vi "Main.vi"(11 "Module Admin":refnum<class "Delacor_lib_QMH_Module Admin.lvclass">) -> ()   [LabVIEW 2020, in "Config.lvlib"]
doc: "This template is based off of the Queued Message Handler design pattern and the Queued Message Handler project template that ships with LabVIEW.\n\nThe main difference is that the queue is private to this module and communication between modules is performed via Broadcast and Request events.\n\nRequest events are wrapped in public API methods and are handled in the Event Handling Loop (EHL) of this VI. Any module can register for Broadcast events sent by this module. The EHL generates messages based on user interface actions.\n\nThe Message Handling Loop (MHL) processes messages generated by the EHL, or by other messages. The messages are string values, so new messages can be added easily to the Message Cases case structure in the MHL. Each message cluster can also provide an optional value for Message Data, which is a variant that can be converted to whatever message-specific data is required.\n_____\nBased on Delacor QMH Project Template 5.0.0.82."
uses:
  Config.lvlib
  <vilib>/Delacor/Delacor QMH/Libraries/Module Admin_class/Delacor_lib_QMH_Module Admin.lvclass
  Module Data--cluster.ctl
  Stop Argument--cluster.ctl
  <vilib>/Delacor/Delacor QMH/Libraries/Message Queue_class/Delacor_lib_QMH_Message Queue.lvclass/Delacor_lib_QMH_Message Queue.ctl
  <vilib>/Utility/miscctls.llb/LVPointTypeDef.ctl
  <vilib>/Delacor/Delacor QMH/Libraries/Module Admin_class/Delacor_lib_QMH_Module Admin.lvclass/Delacor_lib_QMH_Module Admin.ctl
  <vilib>/Delacor/Delacor QMH/Libraries/Message Queue_class/Delacor_lib_QMH_Enqueue Message (Single).vi
  <vilib>/Delacor/Delacor QMH/Libraries/Module Admin_class/Delacor_lib_QMH_Get External Launch.vi
  <vilib>/Utility/error.llb/Error Cluster From Error Code.vi
  <vilib>/ErrorRing/Error Ring.xnode
  <vilib>/Delacor/Delacor QMH/Libraries/Message Queue_class/Delacor_lib_QMH_Message Queue.lvclass
  Acquisition/Acquisition.lvlib
  Loggin/Loggin.lvlib
panel:
  in  "file name":string
  in  "Config":T1={"sampling info"={"Fs"=1000.0, "#s"=1000.0}, "square wave duty cycle (%)"=50.0, "frequency"=10.0, "amplitude"=1.0, "phase"=0.0, "signal type"=enum."Sine Wave"}
  out "error out":errorcluster
  out "Status":string
  # "Config"
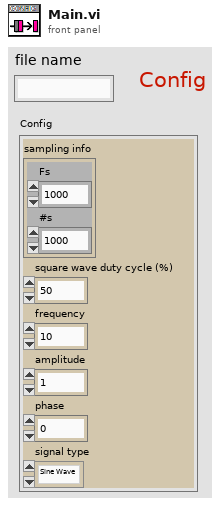
[diagram p1: front panel]
types:
  T1 = cluster{"sampling info":cluster{"Fs":dbl, "#s":dbl}, "square wave duty cycle (%)":dbl, "frequency":dbl, "amplitude":dbl, "phase":dbl, "signal type":enum16{"Sine Wave", "Triangle Wave", "Square Wave", "Sawtooth Wave"}}
  T2 = typedef "Config.lvlib/Request Events--cluster.ctl" = cluster{"Stop Module":refnum<user-event>, "Show Panel":refnum<user-event>, "Hide Panel":refnum<user-event>, "Get Module Execution Status":refnum<user-event>, "Show Diagram":refnum<user-event>}
  T3 = typedef "Config.lvlib/Module Data--cluster.ctl" = cluster{"Status":string}
  T4 = enum32{"invalid lock state", "Not Locked", "Locked (No Password)", "Password-protected"}
  T5 = typedef "Config.lvlib/Stop Argument--cluster.ctl" = cluster{"Origin":string, "Exit via Stop Module Req?":bool, "Wait for Module to stop?":bool}
  T6 = typedef "LVPointTypeDef.ctl" = cluster{"Horizontal":i16, "Vertical":i16}
  T7 = enum32{"Invalid", "Standard", "Closed", "Hidden", "Minimized", "Maximized"}
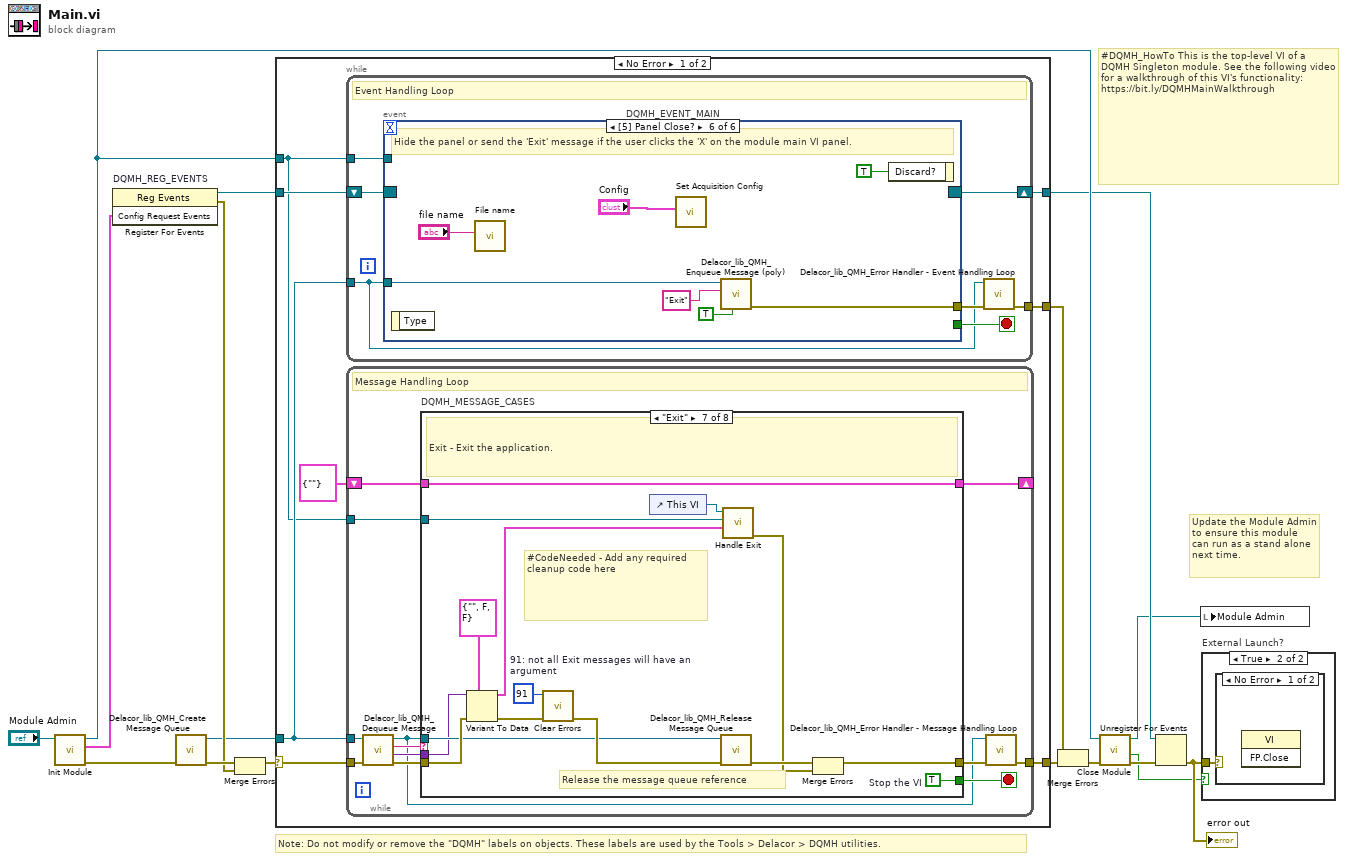
[diagram p0: block diagram]
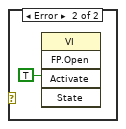
[diagram p3: hidden frame]
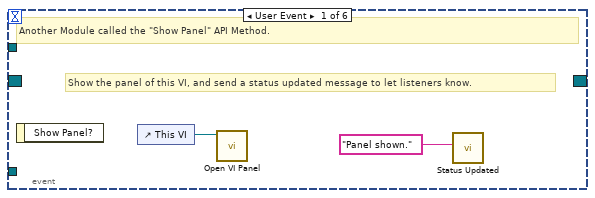
[diagram p4: hidden frame]
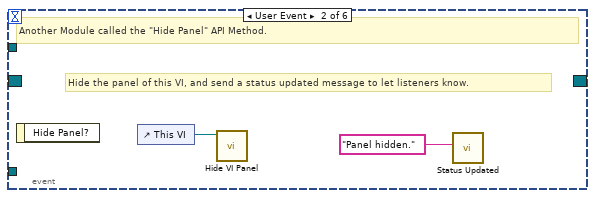
[diagram p5: hidden frame]
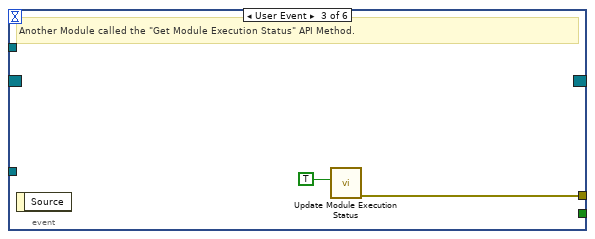
[diagram p6: hidden frame]
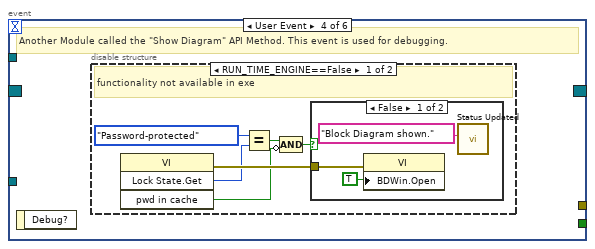
[diagram p7: hidden frame]
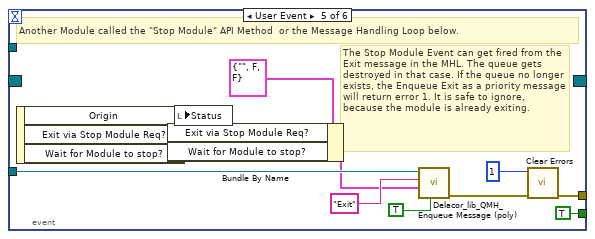
[diagram p10: hidden frame]
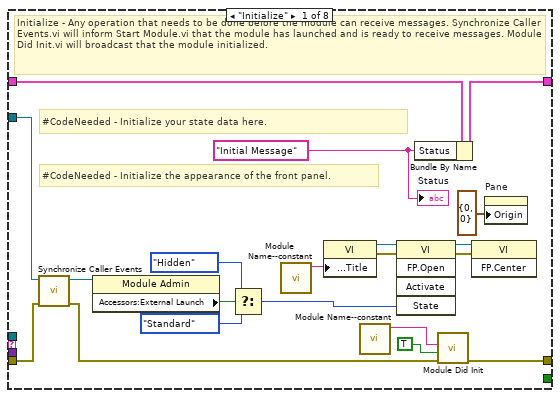
[diagram p11: hidden frame]
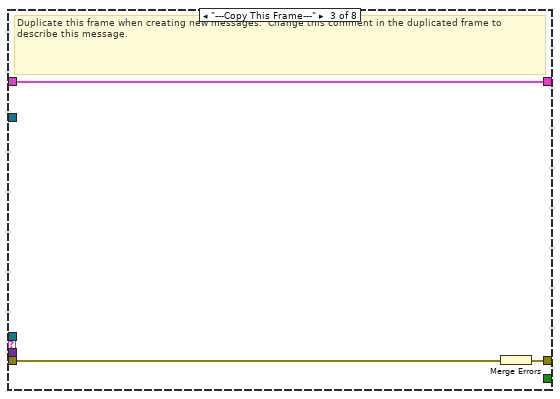
[diagram p13: hidden frame]
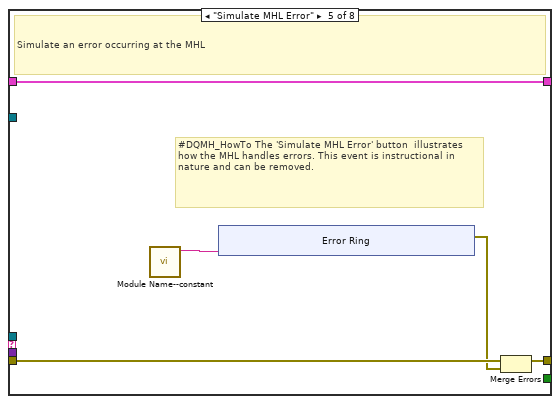
[diagram p15: hidden frame]
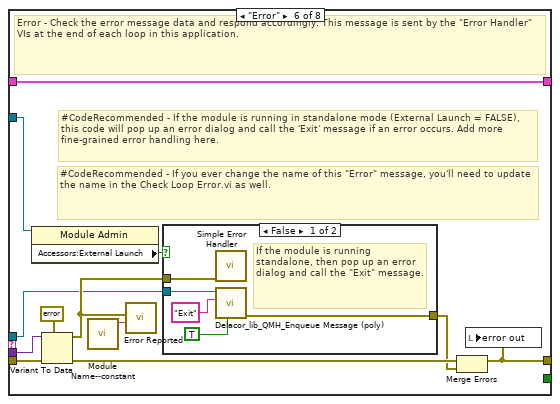
[diagram p16: hidden frame]
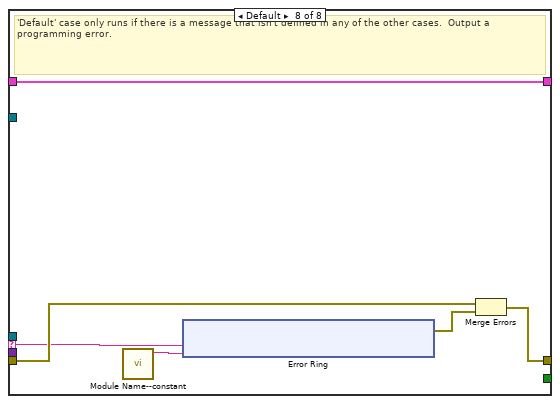
[diagram p18: hidden frame]
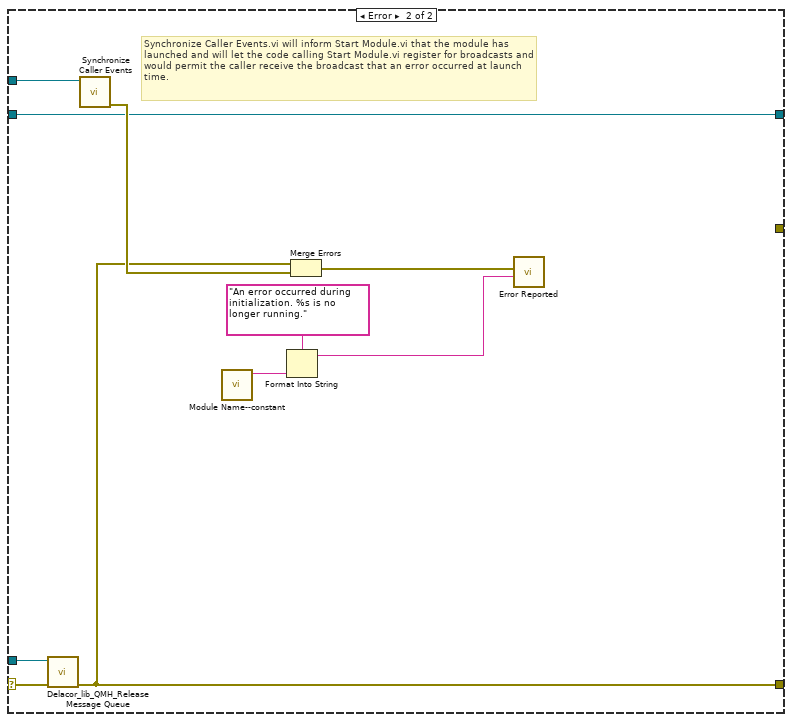
[diagram p19: hidden frame]
diagram:
  # "#DQMH_HowTo This is the top-level VI of a DQMH Singleton module. See the following video for a walkthrough of this VI's functionality: https://bit.ly/DQMHMainWalkthrough"
  # "Note: Do not modify or remove the \"DQMH\" labels on objects. These labels are used by the Tools > Delacor > DQMH utilities."
  # "Update the Module Admin to ensure this module can run as a stand alone next time."
  n1 = call "Init Module.vi"("Singleton Module Admin in"="Module Admin") -> ("error out"=w16:errorcluster, "Config Request Events"=w5:T2, "Singleton Module Admin out"=w8:refnum<class "Delacor_lib_QMH_Module Admin.lvclass">)  [unwired: 8 in]
  n2 = register-events "DQMH_REG_EVENTS"(w5) -> (reference out=w6:refnum<event-registration>, error out=w9:errorcluster)  [unwired: 2 in]
  n3 = call <vilib>:"Delacor_lib_QMH_Create Message Queue.vi"("error in (no error)"=w16) -> ("error out"=w11:errorcluster, "Message Queue"=w4:refnum<class "Delacor_lib_QMH_Message Queue.lvclass">)  [unwired: 9 in]
  n4 = Merge Errors(w11, w9) -> (w10:errorcluster)
  n5 = case shown="No Error" w10 {
    selector: w10 -> [w23 w166]
    tunnel: [w25 w165] -> w17
    tunnel: [w22 w171] -> w7
    tunnel: w6 -> [w20 w171]
    tunnel: w4 -> [w19 w164]
    tunnel: [w24 _] -> w14
    tunnel: w8 -> [w18 w167]
    frame No Error {
      n6 = while {
        tunnel: w19 -> [w26]
        shift-right: [w29] -> w22
        shift-left: w20 -> [w30]
        tunnel: [w31] -> w24
        tunnel: w18 -> [w27]
        stop <- w28 stop-if-true
        # "Event Handling Loop"
        n7 = event "DQMH_EVENT_MAIN" shown="[5] Panel Close?" {
          selector: w30 -> [_ _ _ _ _ _]
          dyn-events: [_ _ _ _ _ _] -> w29
          timeout: _ -> [_ _ _ _ _ _]
          tunnel: [_ _ _ _ TRUE ("Discard?") _] -> w28
          tunnel: w26 -> [_ _ _ _ w55 w64]
          tunnel: [_ _ w38 _ w58 w66] -> w32
          tunnel: w27 -> [_ _ _ _ _ _]
          event User Event {
            # "Show the panel of this VI, and send a status updated message to let listeners know."
            # "Another Module called the \"Show Panel\" API Method."
            n8 = event-data() -> ()  [unwired: 1 in, 1 out]
            n9 = control-ref of="This VI"() -> (w34:refnum<vi>)
            n10 = call "Open VI Panel.vi"("VI"=w34) -> ()  [unwired: 10 in, 1 out]
            n11 = call "Status Updated.vi"("Status"="Panel shown." ("format string")) -> ()  [unwired: 10 in, 1 out]
          }
          event User Event {
            # "Hide the panel of this VI, and send a status updated message to let listeners know."
            # "Another Module called the \"Hide Panel\" API Method."
            n12 = event-data() -> ()  [unwired: 1 in, 1 out]
            n13 = control-ref of="This VI"() -> (w36:refnum<vi>)
            n14 = call "Hide VI Panel.vi"("VI"=w36) -> ()  [unwired: 10 in, 1 out]
            n15 = call "Status Updated.vi"("Status"="Panel hidden." ("format string")) -> ()  [unwired: 10 in, 1 out]
          }
          event User Event {
            # "Another Module called the \"Get Module Execution Status\" API Method."
            n16 = event-data() -> ()  [unwired: 1 in, 1 out]
            n17 = call "Update Module Execution Status.vi"("Running?"=TRUE) -> ("error out"=w38:errorcluster)  [unwired: 10 in]
          }
          event User Event {
            # "Another Module called the \"Show Diagram\" API Method. This event is used for debugging."
            n18 = event-data() -> ()  [unwired: 1 in, 1 out]
            n19 = disable-structure shown="RUN_TIME_ENGINE==False" {
              frame condition #0 (active) {
                # "functionality not available in exe"
                n20 = invoke class="VI" method="Lock State.Get"() -> (error out=w44:errorcluster, "Get Lock State"=w43:T4, "pwd in cache"=w40:bool)  [unwired: 4 in, 1 out]
                n21 = Equal?(x=T4."Password-protected", y=w43) -> (x = y?=w41:bool)
                n22 = Compound Arithmetic op=AND(w41, invert w40) -> (w39:bool)
                n23 = case shown="False" w39 {
                  tunnel: w44 -> [w47 _]
                  frame False {
                    n24 = property class="VI"(error in=w47, "BDWin.Open"=TRUE ("Block Diagram Window:Open")) -> ()  [unwired: 1 in, 2 out]
                    n25 = call "Status Updated.vi"("Status"="Block Diagram shown." ("format string")) -> ()  [unwired: 10 in, 1 out]
                  }
                  frame True {
                    # "Password-protected VI, and the password is not in the cache. Do not show the diagram."
                  }
                }
              }
              frame condition #1 {
              }
            }
          }
          event User Event {
            # "The Stop Module Event can get fired from the Exit message in the MHL. The queue gets destroyed in that case. If the queue no longer exists, the Enqueue Exit as a priority message will return error 1. It is safe to ignore, because the module is already exiting."
            # "Another Module called the \"Stop Module\" API Method  or the Message Handling Loop below."
            n26 = event-data() -> ("Origin"=w54:string, "Exit via Stop Module Req?"=w50:bool, "Wait for Module to stop?"=w49:bool)  [unwired: 1 in]
            n27 = Bundle By Name(cluster=T5 {"Origin"="", "Exit via Stop Module Req?"=FALSE, "Wait for Module to stop?"=FALSE} ("Stop Argument"), "Exit via Stop Module Req?"=w50, "Wait for Module to stop?"=w49) -> (w48:T5)
            n28 = local write "Status"(w54) -> ()
            n29 = call-poly <vilib>:"Delacor_lib_QMH_Enqueue Message (poly).vi"("Priority Message? (F)"=TRUE, "Message Data"=w48, "Message"="Exit", "Message Queue in"=w55) -> ("error out"=w59:errorcluster)  [unwired: 6 in, 1 out]
            n30 = call <vilib>:"Clear Errors.vi"("error in (no error)"=w59, "specific error code to clear (0: all)"=1) -> ("error out"=w58:errorcluster)  [unwired: 4 in, 1 out]
          }
          event Panel Close? {
            # "Hide the panel or send the 'Exit' message if the user clicks the 'X' on the module main VI panel."
            n31 = event-data() -> ()  [unwired: 1 in, 1 out]
            n32 = call "File name.vi"("file name"="file name") -> ()  [unwired: 10 in, 1 out]
            n33 = call "Set Acquisition Config.vi"("Config"="Config") -> ()  [unwired: 10 in, 1 out]
            n34 = call-poly <vilib>:"Delacor_lib_QMH_Enqueue Message (poly).vi"("Priority Message? (F)"=TRUE, "Message"="Exit", "Message Queue in"=w64) -> ("error out"=w66:errorcluster)  [unwired: 7 in, 1 out]
            n35 = event-data("Discard?"=TRUE ("Discard the event, the MHL is responsible for closing and stopping this VI.")) -> ()  [unwired: 1 in, 1 out]
          }
        }
        n36 = call-dynamic "Delacor_lib_QMH_Error Handler - Event Handling Loop.vi"("error in (no error)"=w32, "Message Queue in"=w26) -> ("dup error in"=w31:errorcluster)  [unwired: 8 in, 1 out]
      }
      n37 = while {
        tunnel: w19 -> [w69]
        shift-right: [w73] -> _
        shift-left: T3 {"Status"=""} ("Data Cluster") -> [w74]
        tunnel: w23 -> [w77]
        tunnel: [w75] -> w25
        tunnel: w18 -> [w67]
        stop <- w72 stop-if-true
        # "Message Handling Loop"
        n38 = call-dynamic "Delacor_lib_QMH_Dequeue Message.vi"("error in (no error)"=w77, "Message Queue in"=w69) -> ("error out"=w76:errorcluster, "Message Data"=w70:variant, "Message"=w71:string, "Message Queue out"=w68:refnum<class "Delacor_lib_QMH_Message Queue.lvclass">)  [unwired: 6 in]
        n39 = case "DQMH_MESSAGE_CASES" shown="\"Exit\"" w71 {
          selector: w71 -> [_ _ _ _ _ _ _ w151]
          tunnel: w68 -> [_ _ _ _ _ w121 w143 _]
          tunnel: w76 -> [w96 w100 w103 w105 w110 w128 w149 w153]
          tunnel: [w94 w100 w102 w105 w109 w124 w146 w154] -> w78
          tunnel: w74 -> [w85 w99 w101 w104 w107 w123 w142 w152]
          tunnel: [w84 w99 w101 w104 w107 w123 w142 w152] -> w73
          tunnel: [_ _ _ _ _ _ w141 _] -> w72
          tunnel: w70 -> [_ _ _ _ _ w122 w140 _]
          tunnel: w67 -> [w86 _ _ _ _ w120 w135 _]
          frame "Initialize" {
            w79 = "Initial Message" ("Initial Message")
            # "#CodeNeeded - Initialize the appearance of the front panel."
            # "#CodeNeeded - Initialize your state data here."
            # "Initialize - Any operation that needs to be done before the module can receive messages. Synchronize Caller Events.vi will inform Start Module.vi that the module has launched and is ready to receive messages. Module Did Init.vi will broadcast that the module initialized."
            n40 = call "Synchronize Caller Events.vi"("error in (no error)"=w96, "Singleton Module Admin in"=w86) -> ("error out"=w95:errorcluster, "Singleton Module Admin out"=w81:refnum<class "Delacor_lib_QMH_Module Admin.lvclass">)  [unwired: 8 in]
            n41 = property class="Module Admin"(reference=w81) -> ("Accessors:External Launch"=w90:bool)  [unwired: 1 in, 2 out]
            n42 = Select(t=T7."Hidden" ("State"), s=w90, f=T7."Standard" ("State")) -> (s? t:f=w87:T7)
            n43 = call "Module Name--constant.vi"() -> ("Module Name"=w93:string)  [unwired: 11 in]
            n44 = property class="VI"("Front Panel.Title"=w93) -> (reference out=w92:refnum<vi>, error out=w98:errorcluster)  [unwired: 2 in]
            n45 = call "Module Name--constant.vi"() -> ("Module Name"=w82:string)  [unwired: 11 in]
            n46 = invoke class="VI" method="FP.Open"(reference=w92, error in=w98, "State"=w87) -> (reference out=w91:refnum<vi>, error out=w97:errorcluster)  [unwired: 2 in, 3 out]
            n47 = Bundle By Name(cluster=w85, "Status"=w79) -> (w84:T3)
            n48 = call "Module Did Init.vi"("error in (no error)"=w95, "Initialized?"=TRUE, "Origin"=w82) -> ("error out"=w94:errorcluster)  [unwired: 8 in]
            n49 = invoke class="VI" method="FP.Center"(reference=w91, error in=w97) -> ()  [unwired: 1 in, 3 out]
            n50 = property on="Pane" class="Pane"("Origin"=T6 {"Horizontal"=0, "Vertical"=0}) -> ()  [unwired: 2 in, 2 out]
            "Status" <- w79
          }
          frame "--- Module Specific ---" {
            # "Separator -- The following cases handle messages specific to this Module."
          }
          frame "---Copy This Frame---" {
            # "Duplicate this frame when creating new messages.  Change this comment in the duplicated frame to describe this message."
            n51 = Merge Errors(w103) -> (w102:errorcluster)
          }
          frame "--- Exit and Error Handling---" {
            # "Separator - The following cases handle errors and exit messages."
          }
          frame "Simulate MHL Error" {
            # "#DQMH_HowTo The 'Simulate MHL Error' button  illustrates how the MHL handles errors. This event is instructional in nature and can be removed."
            # "Simulate an error occurring at the MHL"
            n52 = call "Module Name--constant.vi"() -> ("Module Name"=w106:string)  [unwired: 11 in]
            n53 = xnode "Error Ring"("parameter 0"=w106) -> ("error out"=w108:errorcluster)
            n54 = Merge Errors(w110, w108) -> (w109:errorcluster)
          }
          frame "Error" {
            # "#CodeRecommended - If you ever change the name of this \"Error\" message, you'll need to update the name in the Check Loop Error.vi as well."
            # "#CodeRecommended - If the module is running in standalone mode (External Launch = FALSE), this code will pop up an error dialog and call the 'Exit' message if an error occurs. Add more fine-grained error handling here."
            # "Error - Check the error message data and respond accordingly. This message is sent by the \"Error Handler\" VIs at the end of each loop in this application."
            n55 = property class="Module Admin"(reference=w120) -> ("Accessors:External Launch"=w119:bool)  [unwired: 1 in, 2 out]
            n56 = Variant To Data(error in=w128, type=errorcluster {"status"=FALSE, "code"=0, "source"=""} ("error constant"), Variant=w122) -> (data=w129:errorcluster, error out=w126:errorcluster)
            n57 = call "Module Name--constant.vi"() -> ("Module Name"=w118:string)  [unwired: 11 in]
            n58 = call "Error Reported.vi"("Additional Information"=w118, "Error"=w129) -> ()  [unwired: 9 in, 1 out]
            n59 = case shown="False" w119 {
              tunnel: [w134 _] -> w125
              tunnel: w121 -> [w132 _]
              tunnel: w129 -> [w133 _]
              frame False {
                # "If the module is running standalone, then pop up an error dialog and call the \"Exit\" message."
                n60 = call <vilib>:"Simple Error Handler.vi"("error in (no error)"=w133) -> ()  [unwired: 4 in, 5 out]
                n61 = call-poly <vilib>:"Delacor_lib_QMH_Enqueue Message (poly).vi"("Priority Message? (F)"=TRUE, "Message"="Exit", "Message Queue in"=w132) -> ("error out"=w134:errorcluster)  [unwired: 7 in, 1 out]
              }
              frame True {
                # "If the module was launched externally, calling the Error Reported broadcast VI is the only action performed by the \"Error\" message. The module's caller can then process the error appropriately."
              }
            }
            n62 = Merge Errors(w126, w125) -> (w124:errorcluster)
            n63 = local write "error out"(w124) -> ()
          }
          frame "Exit" {
            w139 = 91  # 91: not all Exit messages will have an argument
            w141 = TRUE  # Stop the VI
            # "Release the message queue reference"
            # "#CodeNeeded - Add any required cleanup code here"
            # "Exit - Exit the application."
            n64 = Variant To Data(error in=w149, type=T5 {"Origin"="", "Exit via Stop Module Req?"=FALSE, "Wait for Module to stop?"=FALSE} ("Stop Argument"), Variant=w140) -> (data=w137:T5, error out=w145:errorcluster)
            n65 = call <vilib>:"Clear Errors.vi"("error in (no error)"=w145, "specific error code to clear (0: all)"=w139) -> ("error out"=w148:errorcluster)  [unwired: 4 in, 1 out]
            n66 = control-ref of="This VI"() -> (w136:refnum<vi>)
            n67 = call-dynamic "Delacor_lib_QMH_Release Message Queue.vi"("error in (no error)"=w148, "Message Queue"=w143) -> ("error out"=w147:errorcluster)  [unwired: 9 in]
            n68 = call "Handle Exit.vi"("Stop Argument"=w137, "Admin in"=w135, "VI reference"=w136) -> ("error out"=w144:errorcluster)  [unwired: 7 in, 1 out]
            n69 = Merge Errors(w147, w144) -> (w146:errorcluster)
          }
          frame Default {
            # "'Default' case only runs if there is a message that isn't defined in any of the other cases.  Output a programming error."
            n70 = call "Module Name--constant.vi"() -> ("Module Name"=w150:string)  [unwired: 11 in]
            n71 = xnode "Error Ring"("parameter 0"=w151, "parameter 1"=w150) -> ("error out"=w155:errorcluster)
            n72 = Merge Errors(w153, w155) -> (w154:errorcluster)
          }
        }
        n73 = call-dynamic "Delacor_lib_QMH_Error Handler - Message Handling Loop.vi"("error in (no error)"=w78, "Message Queue in"=w68) -> ("dup error in"=w75:errorcluster)  [unwired: 8 in, 1 out]
      }
    }
    frame Error {
      # "Synchronize Caller Events.vi will inform Start Module.vi that the module has launched and will let the code calling Start Module.vi register for broadcasts and would permit the caller receive the broadcast that an error occurred at launch time."
      n74 = call-dynamic "Delacor_lib_QMH_Release Message Queue.vi"("error in (no error)"=w166, "Message Queue"=w164) -> ("error out"=w165:errorcluster)  [unwired: 9 in]
      n75 = call "Synchronize Caller Events.vi"("Singleton Module Admin in"=w167) -> ("error out"=w172:errorcluster)  [unwired: 9 in, 1 out]
      n76 = call "Module Name--constant.vi"() -> ("Module Name"=w170:string)  [unwired: 11 in]
      n77 = Format Into String(format string="An error occurred during initialization. %s is no longer running.", w170) -> (resulting string=w168:string)  [unwired: 2 in, 1 out]
      n78 = Merge Errors(w165, w172) -> (w173:errorcluster)
      n79 = call "Error Reported.vi"("Additional Information"=w168, "Error"=w173) -> ()  [unwired: 9 in, 1 out]
    }
  }
  n80 = Merge Errors(w14, w17) -> (w13:errorcluster)
  n81 = call "Close Module.vi"("error in (no error)"=w13, "Module Admin in"=w8) -> ("error out"=w15:errorcluster, "External Launch"=w1:bool, "Module Admin out"=w2:refnum<class "Delacor_lib_QMH_Module Admin.lvclass">)  [unwired: 7 in]
  n82 = Unregister For Events(event registration refnum=w7, error in=w15) -> (error out=w12:errorcluster)
  "error out" <- w12
  n83 = local write "Module Admin"(w2) -> ()
  n84 = case "External Launch?" shown="True" w1 {
    tunnel: w12 -> [_ w174]
    frame False {
    }
    frame True {
      n85 = case shown="No Error" w174 {
        frame No Error {
          n86 = invoke class="VI" method="FP.Close"() -> ()  [unwired: 3 in, 3 out]
        }
        frame Error {
          n87 = invoke class="VI" method="FP.Open"("Activate"=TRUE ("Activate?")) -> ()  [unwired: 4 in, 5 out]
        }
      }
    }
  }
